vi "M03 Hybrid Car.vi"(11 "EV3 in":T1) -> (1 "Angle out":sgl, 3 "EV3 out":T1)   [LabVIEW 2016]
uses:
  <vilib>/NXT/Subs/LVHSConnector.ctl
  <vilib>/NXT/LegoClasses/BrickReference/BrickReference.lvclass
  <vilib>/NXT/Dual Mode Library/Waits/Wait_Num.vi
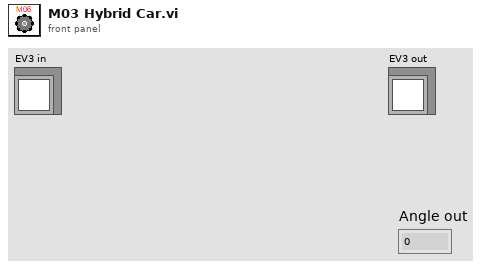
[diagram p1: front panel]
types:
  T1 = typedef "LVHSConnector.ctl" = refnum<class "BrickReference.lvclass">
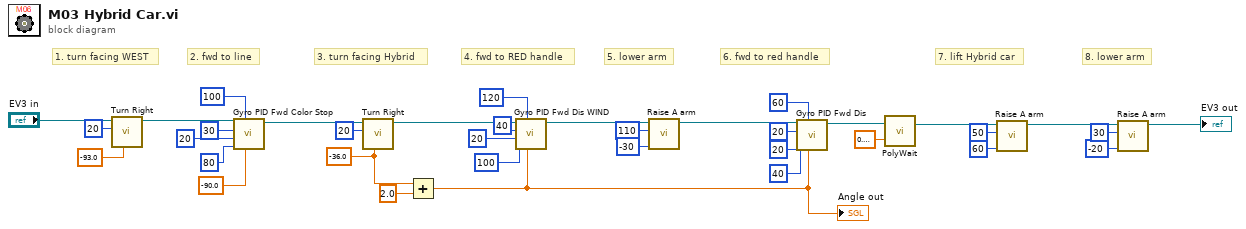
[diagram p0: block diagram]
diagram:
  w22 = sgl -36.0 ("Turning angle")
  # "8. lower arm"
  # "7. lift Hybrid car"
  # "6. fwd to red handle"
  # "5. lower arm"
  # "4. fwd to RED handle"
  # "3. turn facing Hybrid"
  # "2. fwd to line"
  # "1. turn facing WEST"
  n1 = call "Turn Right.vi"("Turning angle"=sgl -93.0, "Motor B (right)"=i8 20, "EV3 in"="EV3 in") -> ("EV3 out"=w34:T1)  [unwired: 8 in]
  n2 = call "Gyro PID Fwd Color Stop.vi"("Target angle"=sgl -90.0, "Threshold to Color"=100, "Threshold to slow"=80, "Min. speed"=20, "Max. speed"=30, "EV3 in"=w34) -> ("EV3 out"=w20:T1)  [unwired: 5 in]
  n3 = call "Turn Right.vi"("Turning angle"=w22, "Motor B (right)"=i8 20, "EV3 in"=w20) -> ("EV3 out"=w26:T1)  [unwired: 8 in]
  n4 = Add(x=w22, y=sgl 2.0) -> (x+y=w8:sgl)
  "Angle out" <- w8
  n5 = call "Gyro PID Fwd Dis WIND.vi"("Target angle"=w8, "Threshold to stop"=120 ("Stop rotation"), "Threshold to slow"=100 ("Threshold to De-acc"), "Higher speed"=20, "Max. speed"=40 ("Acc"), "EV3 in"=w26) -> ("EV3 out"=w14:T1)  [unwired: 5 in]
  n6 = call "Raise A arm.vi"("Power"=i8 -30, "Rotation"=110, "EV3 in"=w14) -> ("EV3 out"=w11:T1)  [unwired: 8 in]
  n7 = call "Gyro PID Fwd Dis.vi"("Target angle"=w8, "Threshold to stop"=60, "Threshold to slow"=40, "Min. speed"=20, "Max. speed"=20, "EV3 in"=w11) -> ("EV3 out"=w6:T1)  [unwired: 5 in]
  n8 = call-poly <vilib>:"PolyWait.vi"("Time (1 sec)"=sgl 0.3, "NXT/EV3"=w6) -> ("NXT/EV3"=w7:T1)  [unwired: 2 in]
  n9 = call "Raise A arm.vi"("Power"=i8 60, "Rotation"=50, "EV3 in"=w7) -> ("EV3 out"=w2:T1)  [unwired: 8 in]
  n10 = call "Raise A arm.vi"("Power"=i8 -20, "Rotation"=30, "EV3 in"=w2) -> ("EV3 out"=→"EV3 out":T1)  [unwired: 8 in]
